vi "DashboardSelectAuto.vi"(0 "Table Prefix":string="330AutonomousSelector", 1 "Autonomous Mode Ring":refnum<vi>) -> ()   [LabVIEW 2014, in "BB_AutonomousSelector.lvlib"]
doc: "Reads the list of Autonomous modes published by the Robot (using the Add Autonomous Mode(s) VIs). Displays them on the referenced menu ring, and allows the user to select a mode and sends the selected mode back to the Robot.\n\n<B>Table Prefix</B> The Sub Table in Network Tables. The data will be stored in /SmartDashboard/<Table Prefix>\n<B>Autonomous Mode Ring</B> A reference to the Menu Ring to use for Autonomous Mode Selection.\n\nThis VI is implemented as a loop. It should be placed in the top level of Dashboard Main, not in any other loop."
uses:
  BB_AutonomousSelector.lvlib
panel:
  in  "Ring":u16(ring)
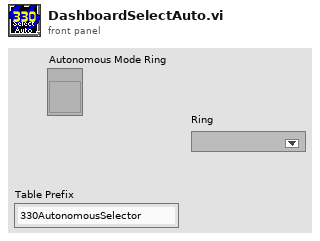
[diagram p1: front panel]
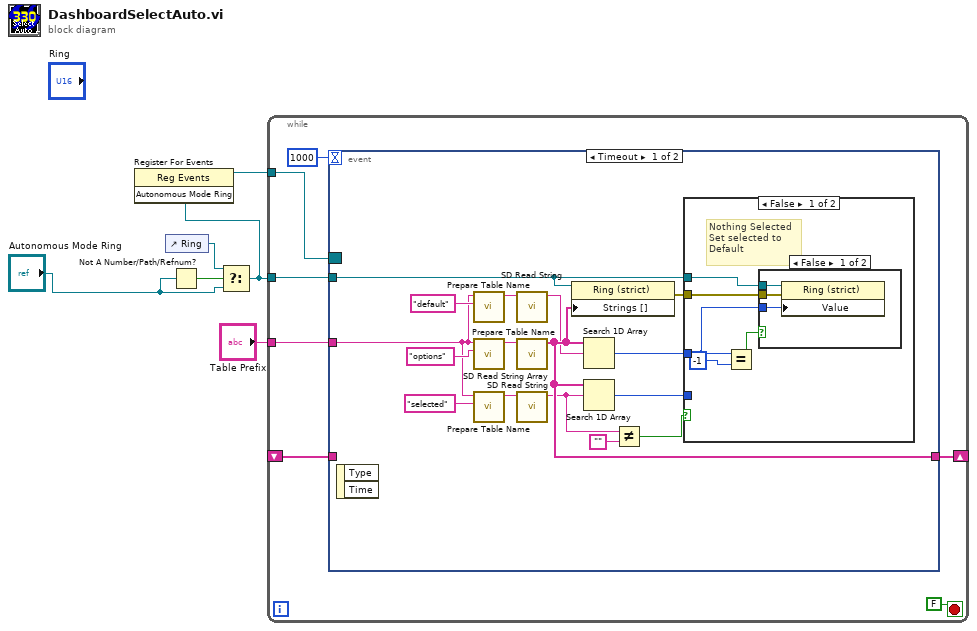
[diagram p0: block diagram]
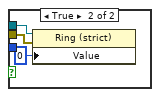
[diagram p2: hidden frame]
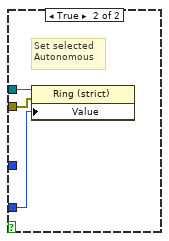
[diagram p3: hidden frame]
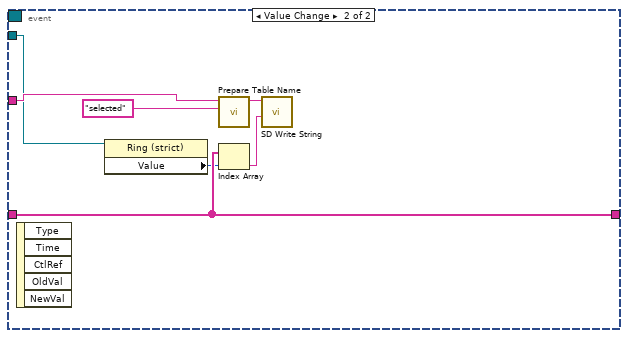
[diagram p4: hidden frame]
diagram:
  n1 = control-ref of="Ring"() -> (w5:refnum<vi>)
  n2 = Not A Number/Path/Refnum?(number/path/refnum="Autonomous Mode Ring") -> (NaN/Path/Refnum?=w4:bool)
  n3 = Select(t=w5, s=w4, f="Autonomous Mode Ring") -> (s? t:f=w2:refnum<vi>)
  n4 = register-events(w2) -> (reference out=w1:refnum<event-registration>)  [unwired: 2 in, 1 out]
  n5 = while {
    shift-right: [w12] -> _
    shift-left: _ -> [w11]
    tunnel: "Table Prefix" -> [w9]
    tunnel: w2 -> [w8]
    tunnel: w1 -> [w7]
    stop <- FALSE stop-if-true
    n6 = event shown="[0] Timeout" {
      selector: w7 -> [_ _]
      dyn-events: _ -> [_ _]
      timeout: 1000 -> [_ _]
      tunnel: [w25 w50] -> w12
      tunnel: w11 -> [_ w50]
      tunnel: w9 -> [w15 w48]
      tunnel: w8 -> [w14 w44]
      event Timeout {
        n7 = event-data() -> ()  [unwired: 1 in, 2 out]
        n8 = call <vilib>:"Prepare Table Name.vi"("Name"="default", "Table Prefix"=w15) -> ("Prefixed Name"=w18:string)  [unwired: 9 in]
        n9 = call <vilib>:"Prepare Table Name.vi"("Name"="options", "Table Prefix"=w15) -> ("Prefixed Name"=w20:string)  [unwired: 9 in]
        n10 = call <vilib>:"Prepare Table Name.vi"("Name"="selected", "Table Prefix"=w15) -> ("Prefixed Name"=w16:string)  [unwired: 9 in]
        n11 = call <vilib>:"SD Read String.vi"("Name"=w18) -> ("String"=w22:string)  [unwired: 8 in, 2 out]
        n12 = call <vilib>:"SD Read String Array.vi"("Name"=w20) -> ("String Array"=w25:string[])  [unwired: 9 in, 1 out]
        n13 = call <vilib>:"SD Read String.vi"("Name"=w16) -> ("String"=w24:string)  [unwired: 8 in, 2 out]
        n14 = property on="Property Node" class="Ring (strict)"(reference=w14, "Strings []"=w25) -> (error out=w29:errorcluster)  [unwired: 1 in, 1 out]
        n15 = Search 1D Array(1D array=w25, element=w22) -> (index of element=w26:i32)  [unwired: 1 in]
        n16 = Search 1D Array(1D array=w25, element=w24) -> (index of element=w23:i32)  [unwired: 1 in]
        n17 = Not Equal?(x=w24, y="") -> (x != y?=w27:bool)
        n18 = case shown="False" w27 {
          tunnel: w29 -> [w34 w43]
          tunnel: w26 -> [w32 _]
          tunnel: w23 -> [_ w42]
          tunnel: w14 -> [w33 w41]
          frame False {
            # "Nothing Selected\nSet selected to\nDefault"
            n19 = Equal?(x=w32, y=-1) -> (x = y?=w30:bool)
            n20 = case shown="False" w30 {
              tunnel: w34 -> [w37 w39]
              tunnel: w33 -> [w36 w40]
              tunnel: w32 -> [w35 _]
              frame False {
                n21 = property on="Property Node" class="Ring (strict)"(reference=w36, error in=w37, "Value"=w35) -> ()  [unwired: 2 out]
              }
              frame True {
                n22 = property on="Property Node" class="Ring (strict)"(reference=w40, error in=w39, "Value"=u16 0) -> ()  [unwired: 2 out]
              }
            }
          }
          frame True {
            # "Set selected\nAutonomous"
            n23 = property on="Property Node" class="Ring (strict)"(reference=w41, error in=w43, "Value"=w42) -> ()  [unwired: 2 out]
          }
        }
      }
      event Value Change {
        n24 = event-data() -> ()  [unwired: 1 in, 5 out]
        n25 = property class="Ring (strict)"(reference=w44) -> ("Value"=w45:u16)  [unwired: 1 in, 2 out]
        n26 = call <vilib>:"Prepare Table Name.vi"("Name"="selected", "Table Prefix"=w48) -> ("Prefixed Name"=w46:string)  [unwired: 9 in]
        n27 = Index Array(array=w50, index=w45) -> (element=w49:string)
        n28 = call <vilib>:"SD Write String.vi"("String"=w49, "Name"=w46) -> ()  [unwired: 8 in, 2 out]
      }
    }
  }
